vi "XIPIN_AXI_Chip2Chip_Bridge_4_2.vi"   [LabVIEW 2017]
doc: "AXI Chip2Chip Bridge\n------------------------------------\n<b>Need License</b> : No\n<b>Interface</b> : AXI4 AXI4-Stream"
uses:
  <vilib>/rvi/XilinxIP/XIPIN_XNode/niFpgaXIPIN.xnode
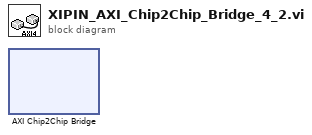
[diagram p0: block diagram]
diagram:
  n1 = xnode ("AXI Chip2Chip Bridge")() -> ()
